vi "testSUBVIS_TOBEREPLACED.vi"(6 "ClassName":string, 9 "Data out":string[](array[string]), 10 "Data out 2":string[](array[string]), 11 "Device space Variable":string) -> (2 "index of element":i32, 3 "delimited string":string)   [LabVIEW 2013]
uses:
  <userlib>/_OpenG.lib/array/array.llb/Index 1D Array Elements (String)__ogtk.vi
panel:
  out "delimited string 2":string
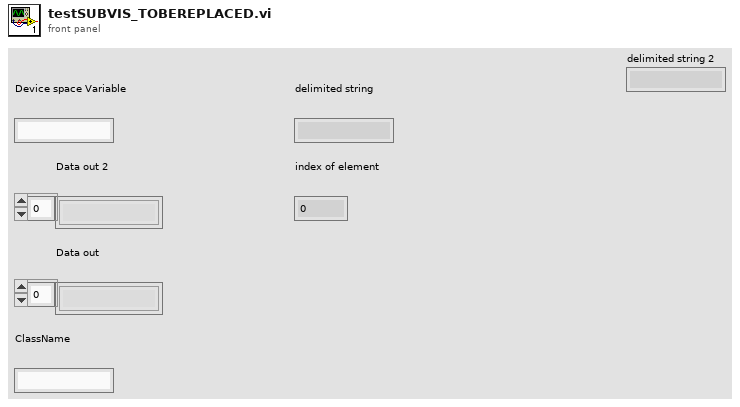
[diagram p1: front panel]
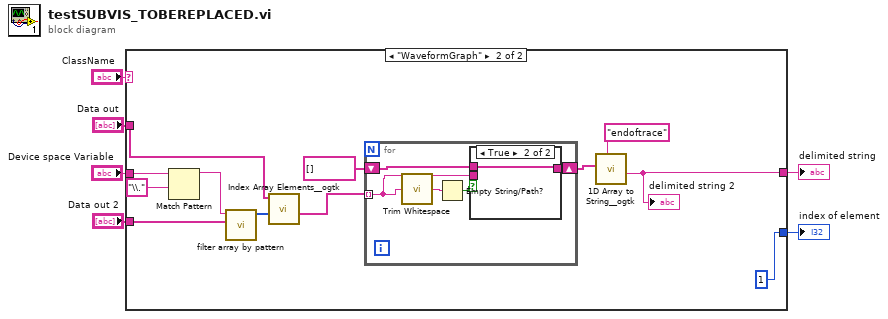
[diagram p0: block diagram]
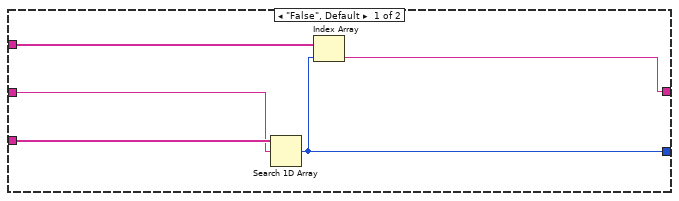
[diagram p2: hidden frame]
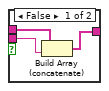
[diagram p3: hidden frame]
diagram:
  n1 = case shown="\"WaveformGraph\"" "ClassName" {
    tunnel: "Data out 2" -> [w11 w18]
    tunnel: "Device space Variable" -> [w10 w22]
    tunnel: "Data out" -> [w9 w21]
    tunnel: [w8 w15] -> w6
    tunnel: [w7 1 ("index of element")] -> w5
    frame "False", Default {
      n2 = Search 1D Array(1D array=w11, element=w10) -> (index of element=w7:i32)  [unwired: 1 in]
      n3 = Index Array(array=w9, index=w7) -> (element=w8:string)
    }
    frame "WaveformGraph" {
      n4 = Match Pattern(string=w22, regular expression="\\.") -> (before substring=w17:string)  [unwired: 1 in, 3 out]
      n5 = call "filter array by pattern.vi"("Array In"=w18, "Pattern In"=w17) -> ("Filtered Array"=w16:i32[])  [unwired: 9 in]
      n6 = call-poly <userlib>:"Index Array Elements__ogtk.vi"("indices"=w16, "array"=w21) -> ("elements"=w14:string[])  [unwired: 9 in]
      n7 = for {
        tunnel: w14 -> [w26] mode=indexing
        shift-right: [w25] -> w12
        shift-left: string[] [] -> [w24]
        n8 = call <vilib>:"Trim Whitespace.vi"("string"=w26) -> ("trimmed string"=w27:string)  [unwired: 1 in]
        n9 = Empty String/Path?(string/path=w27) -> (empty?=w28:bool)
        n10 = case shown="True" w28 {
          tunnel: w26 -> [w31 _]
          tunnel: [w30 w32] -> w25
          tunnel: w24 -> [w29 w32]
          frame False {
            n11 = Build Array (concatenate)(w29, w31) -> (w30:string[])
          }
          frame True {
          }
        }
      }
      n12 = call <userlib>:"1D Array to String__ogtk.vi"("delimiter (Tab)"="endoftrace", "Array of Strings"=w12) -> ("delimited string"=w15:string)  [unwired: 9 in]
      "delimited string 2" <- w15
    }
  }
  "delimited string" <- w6
  "index of element" <- w5
